vi "File_Names_From_Body.vi"(8 "Error In":errorcluster, 11 "Body":string) -> (0 "Error OUt":errorcluster, 3 "File Names":string[](array[string]))   [LabVIEW 2017]
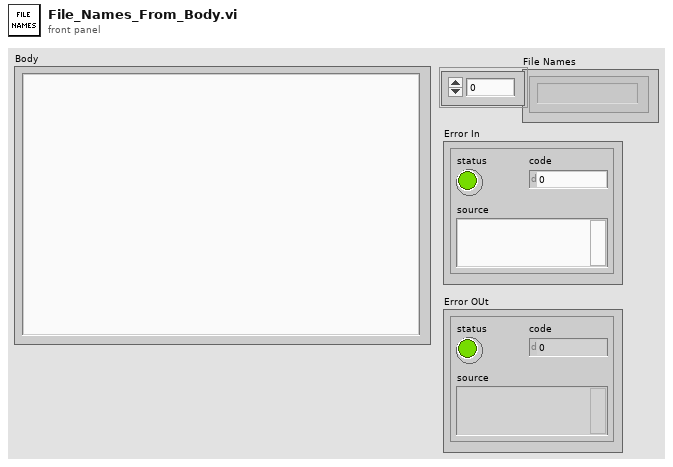
[diagram p1: front panel]
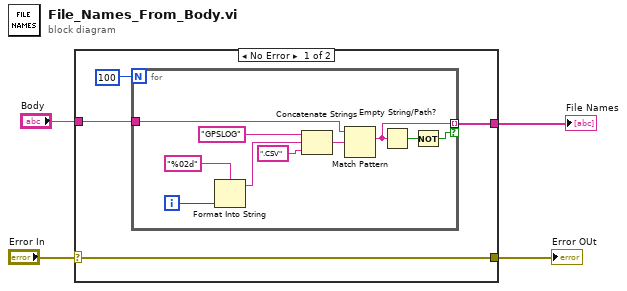
[diagram p0: block diagram]
diagram:
  n1 = case shown="No Error" "Error In" {
    selector: "Error In" -> [w5 w19]
    tunnel: [w8 _] -> w4
    tunnel: "Body" -> [w7 _]
    tunnel: [w5 w19] -> w1
    frame No Error {
      n2 = for {
        N: 100 -> [_]
        tunnel: w7 -> [w18]
        tunnel: [w11] -> w8 mode=indexing if=w9
        i -> [w15]
        n3 = Format Into String(format string="%02d", w15) -> (resulting string=w13:string)  [unwired: 2 in, 1 out]
        n4 = Concatenate Strings("GPSLOG" ("string"), w13, ".CSV" ("string")) -> (w16:string)
        n5 = Match Pattern(string=w18, regular expression=w16) -> (match substring=w11:string)  [unwired: 1 in, 3 out]
        n6 = Empty String/Path?(string/path=w11) -> (empty?=w10:bool)
        n7 = Not(x=w10) -> (.not. x?=w9:bool)
      }
    }
    frame Error {
    }
  }
  "File Names" <- w4
  "Error OUt" <- w1
